vi "h-drive teleop safety.vi"(10 "Gyro Angular Rate":dbl, 11 "Input":dbl) -> (3 "Output":dbl)   [LabVIEW 2014]
uses:
  typedefs/safety data/h-drive teleop safety data.ctl
  global variables/devrefs.vi
  global variables/safeties.vi
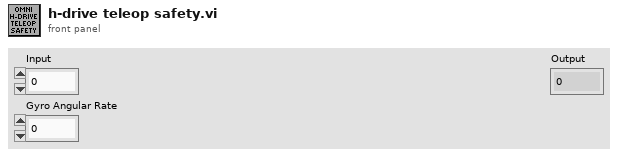
[diagram p1: front panel]
types:
  T1 = typedef "h-drive teleop safety data.ctl" = cluster{"Back Left Encoder Failure":bool, "Back Left No Rate Read":bool, "Back Right Encoder Failure":bool, "Back Right No Rate Read":bool, "Front Left Encoder Failure":bool, "Front Left No Rate Read":bool, "Front Right Encoder Failure":bool, "Front Right No Rate Read":bool, "No Gyro Rate Read":bool, "Gyro Failure":bool}
  T2 = typedef "WPI_EncoderDevRef.ctl" = cluster{"DevStatus":errorcluster, "EncoderIndex":T3, "CounterIndex":T4, "DistancePerCount":dbl, "Decoding Type":T5}
  T3 = typedef "FPGA_EncoderIdx.ctl" = enum8{"Enc 0", "Enc 1", "Enc 2", "Enc 3", "Enc 4", "Enc 5", "Enc 6", "Enc 7", "Invalid"}
  T4 = typedef "FPGA_CounterCtrSystemIndex.ctl" = enum8{"Ctr 0", "Ctr 1", "Ctr 2", "Ctr 3", "Ctr 4", "Ctr 5", "Ctr 6", "Ctr 7", "Invalid"}
  T5 = typedef "WPI_EncoderType.ctl" = enum16{"1x", "2x", "4x"}
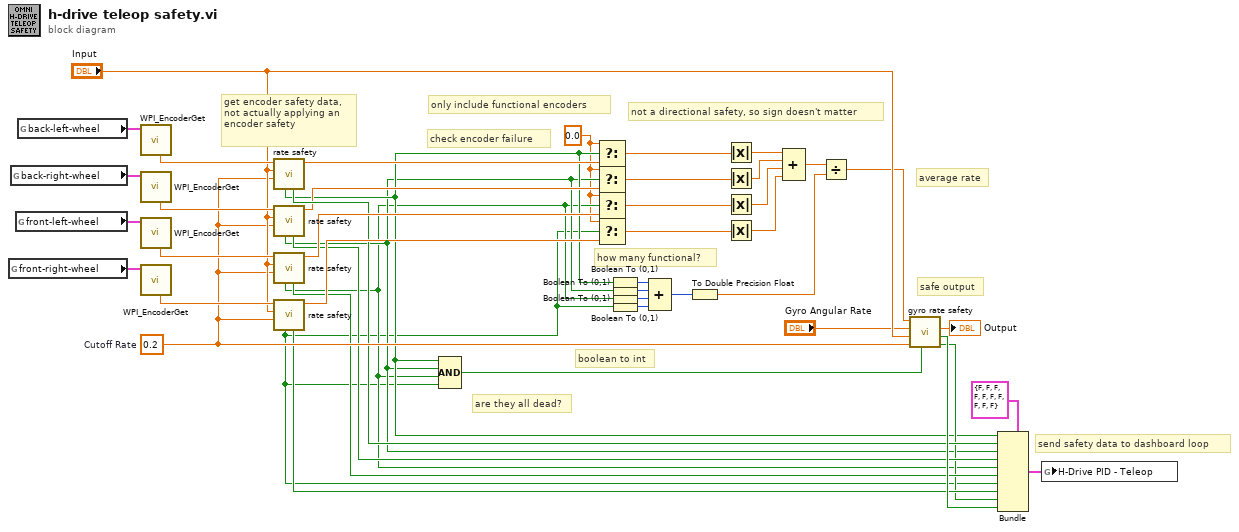
[diagram p0: block diagram]
diagram:
  w7 = 0.0 ("t")
  w27 = 0.2  # Cutoff Rate
  # "boolean to int"
  # "send safety data to dashboard loop"
  # "safe output"
  # "get encoder safety data,\nnot actually applying an \nencoder safety"
  # "check encoder failure"
  # "are they all dead?"
  # "how many functional?"
  # "only include functional encoders"
  # "average rate"
  # "not a directional safety, so sign doesn't matter"
  n1 = global read "devrefs.vi" "front-right-wheel"() -> (w38:T2)
  n2 = global read "devrefs.vi" "back-right-wheel"() -> (w40:T2)
  n3 = global read "devrefs.vi" "front-left-wheel"() -> (w39:T2)
  n4 = global read "devrefs.vi" "back-left-wheel"() -> (w41:T2)
  n5 = call <vilib>:"WPI_EncoderGet.vi"("EncoderDevRef"=w41) -> ("Rate"=w37:dbl)  [unwired: 5 in, 5 out]
  n6 = call <vilib>:"WPI_EncoderGet.vi"("EncoderDevRef"=w40) -> ("Rate"=w36:dbl)  [unwired: 5 in, 5 out]
  n7 = call <vilib>:"WPI_EncoderGet.vi"("EncoderDevRef"=w39) -> ("Rate"=w35:dbl)  [unwired: 5 in, 5 out]
  n8 = call <vilib>:"WPI_EncoderGet.vi"("EncoderDevRef"=w38) -> ("Rate"=w34:dbl)  [unwired: 5 in, 5 out]
  n9 = call "rate safety.vi"("Cutoff Rate"=w27, "Desired Rate"="Input", "Encoder Rate"=w37) -> ("Encoder Rate Out"=w33:dbl, "No Rate Read"=w22:bool, "Encoder Failure"=w12:bool)  [unwired: 5 in, 1 out]
  n10 = call "rate safety.vi"("Cutoff Rate"=w27, "Desired Rate"="Input", "Encoder Rate"=w36) -> ("Encoder Rate Out"=w14:dbl, "No Rate Read"=w21:bool, "Encoder Failure"=w11:bool)  [unwired: 5 in, 1 out]
  n11 = call "rate safety.vi"("Cutoff Rate"=w27, "Desired Rate"="Input", "Encoder Rate"=w35) -> ("Encoder Rate Out"=w32:dbl, "No Rate Read"=w20:bool, "Encoder Failure"=w10:bool)  [unwired: 5 in, 1 out]
  n12 = call "rate safety.vi"("Cutoff Rate"=w27, "Desired Rate"="Input", "Encoder Rate"=w34) -> ("Encoder Rate Out"=w31:dbl, "No Rate Read"=w19:bool, "Encoder Failure"=w8:bool)  [unwired: 5 in, 1 out]
  n13 = Compound Arithmetic op=AND(w12, w11, w10, w8) -> (w23:bool)
  n14 = Select(t=w7, s=w12, f=w33) -> (s? t:f=w16:dbl)
  n15 = Select(t=w7, s=w11, f=w14) -> (s? t:f=w15:dbl)
  n16 = Select(t=w7, s=w10, f=w32) -> (s? t:f=w13:dbl)
  n17 = Select(t=w7, s=w8, f=w31) -> (s? t:f=w9:dbl)
  n18 = Boolean To (0,1)(Boolean=w12) -> (0, 1=w6:i16)
  n19 = Boolean To (0,1)(Boolean=w11) -> (0, 1=w5:i16)
  n20 = Boolean To (0,1)(Boolean=w10) -> (0, 1=w4:i16)
  n21 = Boolean To (0,1)(Boolean=w8) -> (0, 1=w3:i16)
  n22 = Compound Arithmetic op=ADD(w6, w5, w4, w3) -> (w2:i16)
  n23 = To Double Precision Float(number=w2) -> (double precision float=w1:dbl)
  n24 = Absolute Value(x=w16) -> (abs(x)=w42:dbl)
  n25 = Absolute Value(x=w15) -> (abs(x)=w43:dbl)
  n26 = Absolute Value(x=w13) -> (abs(x)=w44:dbl)
  n27 = Absolute Value(x=w9) -> (abs(x)=w45:dbl)
  n28 = Compound Arithmetic op=ADD(w42, w43, w44, w45) -> (w46:dbl)
  n29 = Divide(x=w46, y=w1) -> (x/y=w29:dbl)
  n30 = call "gyro rate safety.vi"("Encoder Failure"=w23, "Cutoff Rate"=w27, "Input"="Input", "Gyro Angular Rate"="Gyro Angular Rate", "Encoder Rate"=w29) -> ("No Gyro Rate Read"=w18:bool, "Gyro Failure"=w24:bool, "Output"=→"Output":dbl)  [unwired: 3 in, 1 out]
  n31 = Bundle(cluster=T1 {"Back Left Encoder Failure"=FALSE, "Back Left No Rate Read"=FALSE, "Back Right Encoder Failure"=FALSE, "Back Right No Rate Read"=FALSE, "Front Left Encoder Failure"=FALSE, "Front Left No Rate Read"=FALSE, "Front Right Encoder Failure"=FALSE, "Front Right No Rate Read"=FALSE, "No Gyro Rate Read"=FALSE, "Gyro Failure"=FALSE}, "Back Left Encoder Failure"=w12, "Back Left No Rate Read"=w22, "Back Right Encoder Failure"=w11, "Back Right No Rate Read"=w21, "Front Left Encoder Failure"=w10, "Front Left No Rate Read"=w20, "Front Right Encoder Failure"=w8, "Front Right No Rate Read"=w19, "No Gyro Rate Read"=w18, "Gyro Failure"=w24) -> (w25:T1)
  n32 = global write "safeties.vi" "H-Drive PID - Teleop"(w25) -> ()
